vi "get_digital_output_line.vi"(8 "error in (no error)":errorcluster, 11 "DAQmxDigitalOut in":refnum<class "DigitalOutDL110325DAQmx.lvclass">) -> (0 "error out":errorcluster, 2 "digital output line":tag, 3 "DAQmxDigitalOut out":refnum<class "DigitalOutDL110325DAQmx.lvclass">)   [LabVIEW 2010, in "DigitalOutDL110325DAQmx.lvclass"]
uses:
  DigitalOutDL110325DAQmx.lvclass
  DigitalOutDL110325DAQmx.lvclass/DigitalOutDL110325DAQmx.ctl
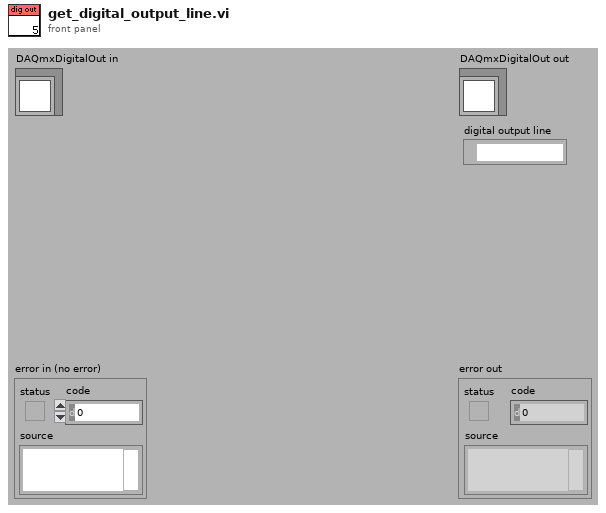
[diagram p1: front panel]
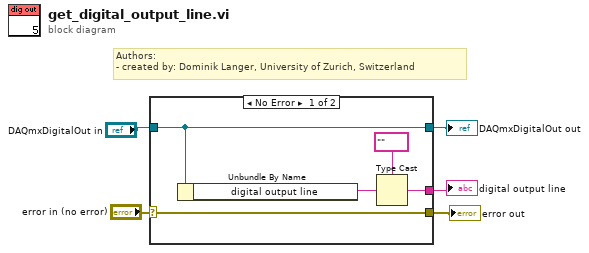
[diagram p0: block diagram]
diagram:
  # "Authors: \n- created by: Dominik Langer, University of Zurich, Switzerland"
  n1 = case shown="No Error" "error in (no error)" {
    selector: "error in (no error)" -> [w10 w12]
    tunnel: [w10 w12] -> w4
    tunnel: [w9 w11] -> w2
    tunnel: "DAQmxDigitalOut in" -> [w9 w11]
    tunnel: [w6 _] -> w1
    frame No Error {
      n2 = Unbundle By Name(w9) -> ("digital output line"=w8:string)
      n3 = Type Cast(type=tag "" ("lines"), x=w8) -> (*(type *) &x=w6:tag)
    }
    frame Error {
    }
  }
  "error out" <- w4
  "DAQmxDigitalOut out" <- w2
  "digital output line" <- w1
